vi "NI Restore Window.vi"(8 "error in (no error)":errorcluster, 11 "window name  (\"\")":string) -> (0 "error out":errorcluster)   [LabVIEW 2018]
doc: "This function will restore the window named in the window name input if the window refnum supplied is invalid, otherwise it uses window refnum to determine which window is restored. If the window cannot be found, an error will be returned."
uses:
  LVWUtil32.dll
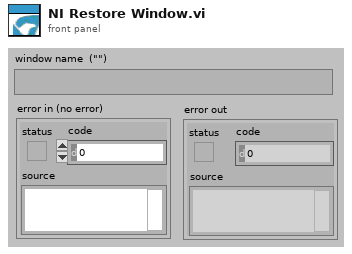
[diagram p1: front panel]
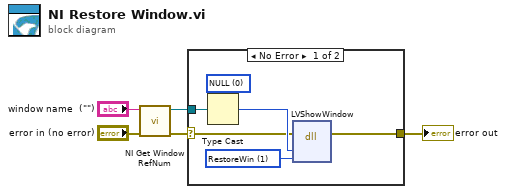
[diagram p0: block diagram]
diagram:
  n1 = call "NI Get Window RefNum.vi"("error in (no error)"="error in (no error)", "window name (\"\")"="window name  (\"\")") -> ("error out"=w1:errorcluster, "window refnum (NaWR)"=w5:refnum<k1>)  [unwired: 8 in]
  n2 = case shown="No Error" w1 {
    selector: w1 -> [w6 w12]
    tunnel: w5 -> [w8 _]
    tunnel: [w7 w12] -> w2
    frame No Error {
      w11 = u8 1 items=["ShowWindow", "RestoreWin"]
      w9 = u32 0 items=["NULL"]
      n3 = Type Cast(type=w9, x=w8) -> (*(type *) &x=w10:u32)
      n4 = dll-call lib="C:/Users/John Gmitter/OneDrive - National Instruments/Projects/Harris FL/Manticore/Harris SW upgrades/Reference Management Server/Generic Reuse/Windows Utilities/lvwutil32.dll" fn="LVShowWindow"(error in=w6, "hWnd"=w10, "function"=w11) -> (error out=w7:errorcluster)  [unwired: 5 in, 1 out]
    }
    frame Error {
    }
  }
  "error out" <- w2
